vi "String_to_UserAccount.vi"(1 "String account":string) -> (0 "Account":T1)   [LabVIEW 2012]
uses:
  typedef/User Accounts.ctl
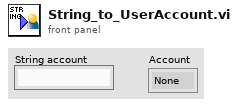
[diagram p1: front panel]
types:
  T1 = typedef "User Accounts.ctl" = enum16{"None", "User", "Admin"}
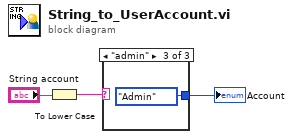
[diagram p0: block diagram]
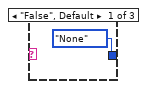
[diagram p2: hidden frame]
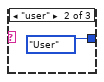
[diagram p3: hidden frame]
diagram:
  n1 = To Lower Case(string="String account") -> (all lower case string=w2:string)
  n2 = case shown="\"admin\"" w2 {
    tunnel: [User_Accounts."None" ("Account 2") User_Accounts."User" ("Account 2") User_Accounts."Admin" ("Account 2")] -> w3
    frame "False", Default {
    }
    frame "user" {
    }
    frame "admin" {
    }
  }
  "Account" <- w3
